vi "Normalize Path String.vi"(3 "Path String":string) -> (1 "Path":path)   [LabVIEW 2020, in "CDM-Config.lvlib"]
uses:
  CDM-Config.lvlib
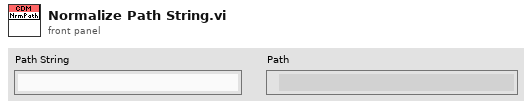
[diagram p1: front panel]
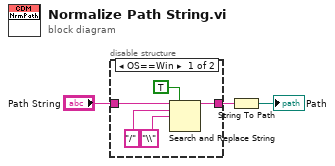
[diagram p0: block diagram]
diagram:
  n1 = disable-structure shown="OS==Win" {
    disable-tunnel: "Path String" -> [w8 _]
    disable-tunnel: [w4 _] -> w2
    frame condition #0 (active) {
      n2 = Search and Replace String(replace all?=TRUE ("replace all? (F)"), input string=w8, search string="/", replace string="\\" ("search string")) -> (result string=w4:string)  [unwired: 4 in, 3 out]
    }
    frame condition #1 {
    }
  }
  n3 = String To Path(string=w2) -> (path=→"Path":path)
